vi "svx_Polar_Draw_Arrow.vi"(4 "shaft rotating direction":u16(ring) items=["CCW", "CW"], 6 "color":u32(colorbox)=10184, 10 "Plot Area:Size":cluster{"Width":u32, "Height":u32}={"Width"=100, "Height"=100}, 11 "Picture in":picture) -> (1 "F/B position":cluster{dbl, dbl}, 2 "Plot Area:Size out":cluster{"Width":u32, "Height":u32}={"Width"=100, "Height"=100}, 3 "Picture out":picture)   [LabVIEW 2017, in "SVX Polar Plot.xctl"]
uses:
  <vilib>/addons/_XControls/Polar Plot/SVX Polar Plot.xctl
panel:
  in  "pen":T1={"Width"=2, "Style"=enum."Solid"}
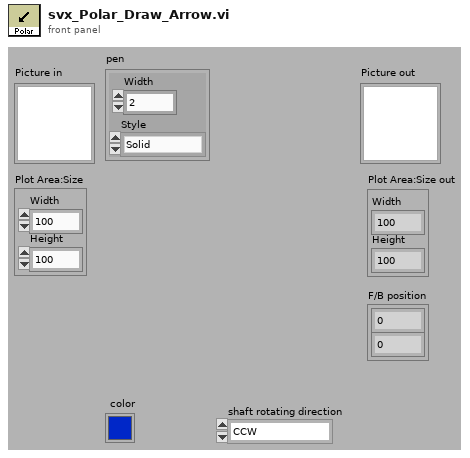
[diagram p1: front panel]
types:
  T1 = cluster{"Width":u16, "Style":enum32{"Solid", "Dash", "Dot", "DashDot", "DashDotDot"}}
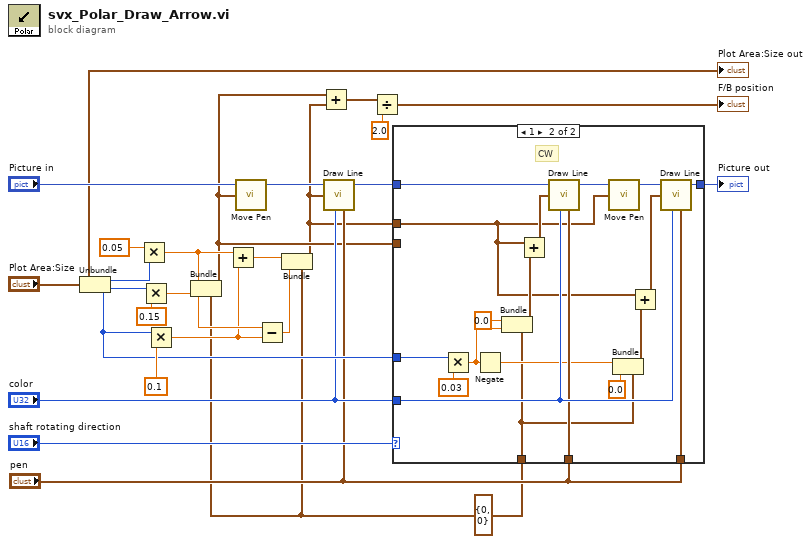
[diagram p0: block diagram]
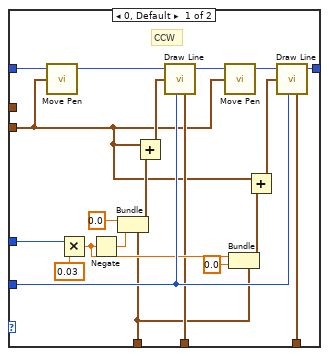
[diagram p2: hidden frame]
diagram:
  w1 = cluster{"x":i16, "y":i16} {"x"=0, "y"=0} ("cluster")
  n1 = Unbundle("Plot Area:Size") -> ("Width"=w21:u32, "Height"=w13:u32)
  n2 = Multiply(x=0.05 ("y"), y=w21) -> (x*y=w19:dbl)
  n3 = Multiply(x=w13, y=0.15) -> (x*y=w17:dbl)
  n4 = Multiply(x=w13, y=0.1) -> (x*y=w16:dbl)
  n5 = Bundle(cluster=w1, "x"=w19, "y"=w17) -> (w6:cluster{"x":i16, "y":i16})
  n6 = Add(x=w19, y=w16) -> (x+y=w15:dbl)
  n7 = call <vilib>:"Move Pen.vi"("new position"=w6, "picture"="Picture in") -> ("new picture"=w24:picture)  [unwired: 3 in]
  n8 = Subtract(x=w17, y=w16) -> (x-y=w14:dbl)
  n9 = Bundle(cluster=w1, "x"=w15, "y"=w14) -> (w5:cluster{"x":i16, "y":i16})
  n10 = Add(x=w6, y=w5) -> (x+y=w3:cluster{"x":i16, "y":i16})
  n11 = call <vilib>:"Draw Line.vi"("picture"=w24, "end point"=w5, "color(black)"="color", "pen"="pen") -> ("new picture"=w7:picture)  [unwired: 5 in]
  n12 = Divide(x=w3, y=2.0) -> (x/y=→"F/B position":cluster{"x":dbl, "y":dbl})
  n13 = case shown="1" "shaft rotating direction" {
    tunnel: w13 -> [w43 w62]
    tunnel: "color" -> [w38 w59]
    tunnel: w6 -> [w26 _]
    tunnel: [w33 w56] -> w11
    tunnel: "pen" -> [w30 w53]
    tunnel: "pen" -> [w29 w52]
    tunnel: w7 -> [w28 w51]
    tunnel: w5 -> [_ w50]
    tunnel: w1 -> [w25 w45]
    frame 0, Default {
      # "CCW"
      n14 = call <vilib>:"Move Pen.vi"("new position"=w26, "picture"=w28) -> ("new picture"=w27:picture)  [unwired: 3 in]
      n15 = Multiply(x=w43, y=0.03) -> (x*y=w37:dbl)
      n16 = Negate(x=w37) -> (-x=w42:dbl)
      n17 = Bundle(cluster=w25, "x"=0.0 ("-x"), "y"=w42) -> (w40:cluster{"x":i16, "y":i16})
      n18 = Add(x=w26, y=w40) -> (x+y=w39:cluster{"x":i16, "y":i16})
      n19 = call <vilib>:"Draw Line.vi"("picture"=w27, "end point"=w39, "color(black)"=w38, "pen"=w30) -> ("new picture"=w32:picture)  [unwired: 5 in]
      n20 = call <vilib>:"Move Pen.vi"("new position"=w26, "picture"=w32) -> ("new picture"=w31:picture)  [unwired: 3 in]
      n21 = Bundle(cluster=w25, "x"=w37, "y"=0.0 ("-x")) -> (w35:cluster{"x":i16, "y":i16})
      n22 = Add(x=w26, y=w35) -> (x+y=w34:cluster{"x":i16, "y":i16})
      n23 = call <vilib>:"Draw Line.vi"("picture"=w31, "end point"=w34, "color(black)"=w38, "pen"=w29) -> ("new picture"=w33:picture)  [unwired: 5 in]
    }
    frame 1 {
      # "CW"
      n24 = Multiply(x=w62, y=0.03) -> (x*y=w49:dbl)
      n25 = Negate(x=w49) -> (-x=w47:dbl)
      n26 = Bundle(cluster=w45, "x"=0.0 ("-x"), "y"=w49) -> (w61:cluster{"x":i16, "y":i16})
      n27 = Add(x=w50, y=w61) -> (x+y=w60:cluster{"x":i16, "y":i16})
      n28 = call <vilib>:"Draw Line.vi"("picture"=w51, "end point"=w60, "color(black)"=w59, "pen"=w53) -> ("new picture"=w55:picture)  [unwired: 5 in]
      n29 = call <vilib>:"Move Pen.vi"("new position"=w50, "picture"=w55) -> ("new picture"=w54:picture)  [unwired: 3 in]
      n30 = Bundle(cluster=w45, "x"=w47, "y"=0.0 ("-x")) -> (w58:cluster{"x":i16, "y":i16})
      n31 = Add(x=w50, y=w58) -> (x+y=w57:cluster{"x":i16, "y":i16})
      n32 = call <vilib>:"Draw Line.vi"("picture"=w54, "end point"=w57, "color(black)"=w59, "pen"=w52) -> ("new picture"=w56:picture)  [unwired: 5 in]
    }
  }
  "Picture out" <- w11
  "Plot Area:Size out" <- "Plot Area:Size"
